vi "Flush Spy Queue.vi"(8 "error in (no error)":errorcluster, 11 "Mock Voltage Output in":refnum<class "Mock Voltage Output.lvclass">) -> (0 "error out":errorcluster, 2 "Setpoints":dbl[](array[numeric]), 3 "Mock Voltage Output out":refnum<class "Mock Voltage Output.lvclass">)   [LabVIEW 2020, in "High Level PSU With Tests.lvlib" / "Mock Voltage Output.lvclass"]
uses:
  Mock Voltage Output.lvclass
  Mock Voltage Output.lvclass/Mock Voltage Output.ctl
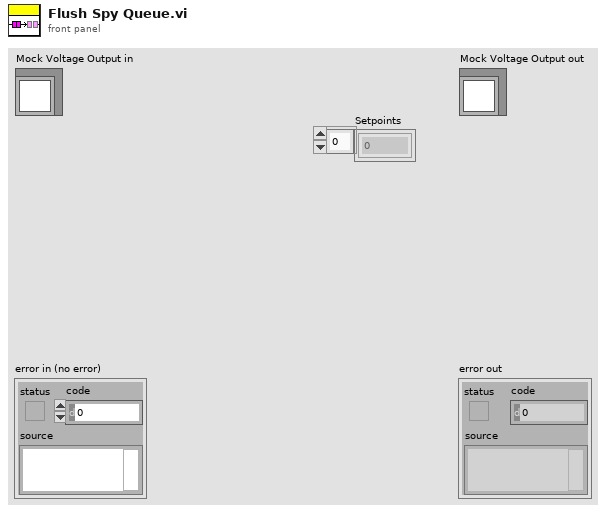
[diagram p1: front panel]
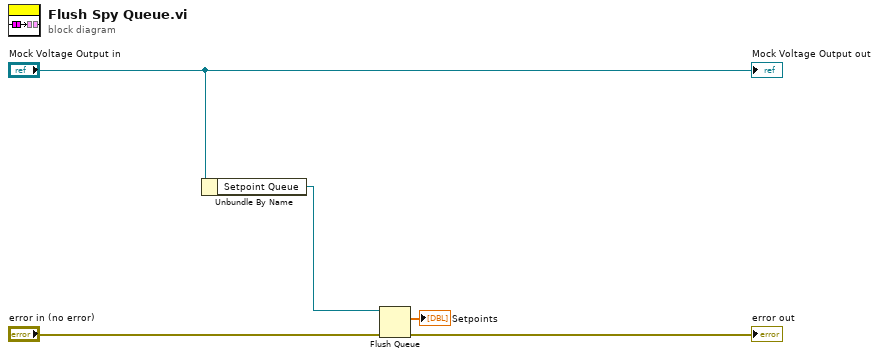
[diagram p0: block diagram]
diagram:
  n1 = Unbundle By Name("Mock Voltage Output in") -> ("Setpoint Queue"=w2:refnum<queue>)
  n2 = Flush Queue(queue=w2, error in (no error)="error in (no error)") -> (remaining elements=→"Setpoints":dbl[], error out=→"error out":errorcluster)  [unwired: 1 out]
  "Mock Voltage Output out" <- "Mock Voltage Output in"
